vi "UART Reading Module.vi"(8 "error in (no error)":errorcluster, 11 "VISA Refnum in":refnum<visa-resource-name>) -> (0 "error out":errorcluster, 2 "Array with 6 col":u8[][](array[numeric]), 3 "VISA resource name out":refnum<visa-resource-name>)   [LabVIEW 2025]
panel:
  # "Inputs"
  # "Outputs"
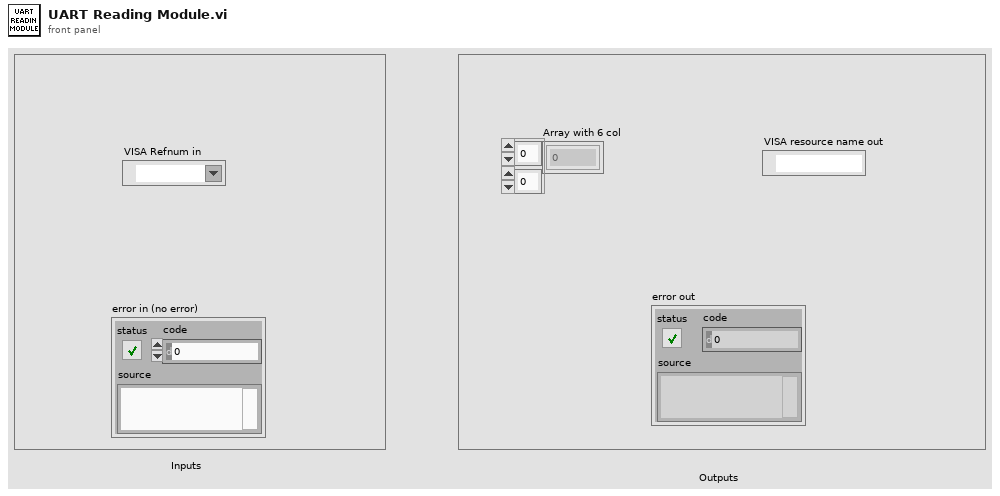
[diagram p1: front panel]
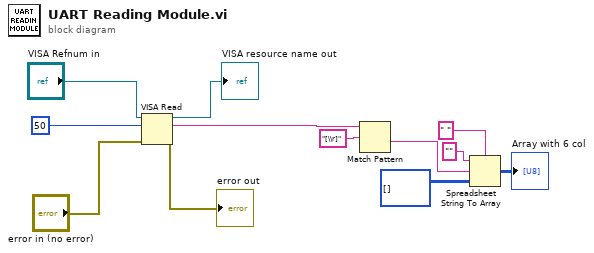
[diagram p0: block diagram]
diagram:
  n1 = VISA Read(VISA resource name="VISA Refnum in", byte count=u32 50, error in (no error)="error in (no error)") -> (VISA resource name out=→"VISA resource name out":refnum<visa-resource-name>, read buffer=w6:string, error out=→"error out":errorcluster)  [unwired: 1 out]
  n2 = Match Pattern(string=w6, regular expression="[\\r]") -> (after substring=w9:string)  [unwired: 1 in, 3 out]
  n3 = Spreadsheet String To Array(delimiter (Tab)=" ", format string="", spreadsheet string=w9, array type (2D Dbl)=u8[][] []) -> (array=→"Array with 6 col":u8[][])
